vi "ASCII Intermittent.vi"() -> ()   [LabVIEW 2019]
uses:
  <vilib>/Instr/_visa.llb/VISA Configure Serial Port (Instr).vi
panel:
  out "read buffer":string
  out "error out":errorcluster
  in  "stop":bool
  in  "VISA resource name":refnum<visa-resource-name>
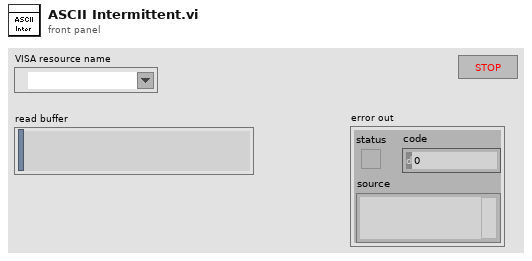
[diagram p1: front panel]
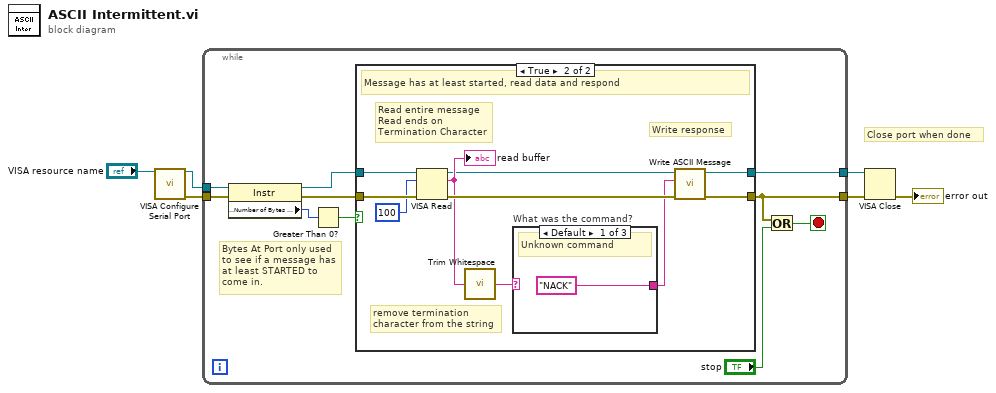
[diagram p0: block diagram]
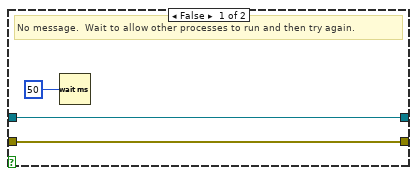
[diagram p2: hidden frame]
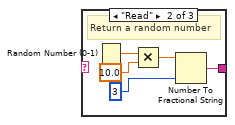
[diagram p3: hidden frame]
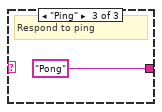
[diagram p4: hidden frame]
diagram:
  # "Close port when done"
  n1 = call-poly "VISA Configure Serial Port"("VISA resource name"="VISA resource name") -> ("VISA resource name out"=w1:refnum<visa-resource-name>, "error out"=w4:errorcluster)  [unwired: 13 in]
  n2 = while {
    tunnel: w4 -> [w16]
    tunnel: w1 -> [w13]
    tunnel: [w9] -> w2
    tunnel: [w14] -> w6
    stop <- w8 stop-if-true
    # "Bytes At Port only used\nto see if a message has\nat least STARTED to\ncome in."
    n3 = property class="Instr"(reference=w13, error in=w16) -> (reference out=w10:refnum<visa-resource-name>, error out=w15:errorcluster, "Serial Settings:Number of Bytes at Serial Port"=w12:u32)
    n4 = Greater Than 0?(x=w12) -> (x > 0?=w11:bool)
    n5 = case shown="True" w11 {
      tunnel: w15 -> [w19 w29]
      tunnel: w10 -> [w18 w26]
      tunnel: [w18 w21] -> w9
      tunnel: [w19 w27] -> w14
      frame False {
        # "No message.  Wait to allow other processes to run and then try again."
        n6 = Wait (ms)(milliseconds to wait=u32 50) -> ()  [unwired: 1 out]
      }
      frame True {
        # "remove termination\ncharacter from the string"
        # "Write response"
        # "Read entire message\nRead ends on\nTermination Character"
        # "Message has at least started, read data and respond"
        n7 = VISA Read(VISA resource name=w26, byte count=u32 100, error in (no error)=w29) -> (VISA resource name out=w23:refnum<visa-resource-name>, read buffer=w24:string, error out=w28:errorcluster)  [unwired: 1 out]
        "read buffer" <- w24
        n8 = call <vilib>:"Trim Whitespace.vi"("string"=w24) -> ("trimmed string"=w20:string)  [unwired: 1 in]
        n9 = case "What was the command?" shown="Default" w20 {
          tunnel: ["NACK" ("write buffer") w31 "Pong" ("write buffer")] -> w22
          frame Default {
            # "Unknown command"
          }
          frame "Read" {
            # "Return a random number"
            n10 = Random Number (0-1)() -> (number: 0 to 1=w35:dbl)
            n11 = Multiply(x=w35, y=10.0) -> (x*y=w33:dbl)
            n12 = Number To Fractional String(number=w33, precision (6)=i16 3) -> (F-format string=w31:string)  [unwired: 2 in]
          }
          frame "Ping" {
            # "Respond to ping"
          }
        }
        n13 = call "Write ASCII Message.vi"("error in"=w28, "Message"=w22, "VISA resource in"=w23) -> ("error out"=w27:errorcluster, "VISA resource out"=w21:refnum<visa-resource-name>)  [unwired: 7 in]
      }
    }
    n14 = Or(x=w14, y="stop") -> (x .or. y?=w8:bool)
  }
  n15 = VISA Close(VISA resource name=w2, error in (no error)=w6) -> (error out=→"error out":errorcluster)
